vi "excel delete worksheet.vi"(8 "error in (no error)":errorcluster, 9 "Name of Worksheet to Delete":string="Sheet1", 10 "New worksheet":string="Intro", 11 "reference":T1) -> (0 "error out":errorcluster, 3 "reference out":T1)   [LabVIEW 2013]
doc: "Make a copy of active sheet. you can specify if the original is the active sheet \nafter the copy or the destination (copied sheet) should be active... \n\nYou need to supply a valid worksheet name (=destination), it should be unique \nwithin the workbook. to get a list of open sheets, use excel info.vi \n \nPhilips Research, COS/TMA"
uses:
  excel.llb/excel Object Reference.ctl
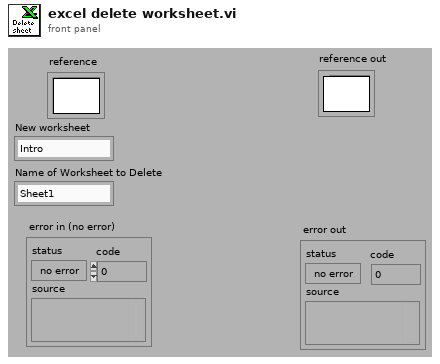
[diagram p1: front panel]
types:
  T1 = typedef "excel Object Reference.ctl" = refnum<k1>
  T2 = typedef "excel Data Members.ctl" = cluster{"Excel._Application":refnum<k7>, "Excel._Workbook":refnum<k7>, "Excel._Worksheet":refnum<k7>, "template?":bool, "location":cluster{"TopLeft":string, "RightBottom":string}, "positioning info":cluster{"direction":enum16{"right", "down"}, "gap":i32}}
  T3 = cluster{"direction":enum16{"right", "down"}, "gap":i32}
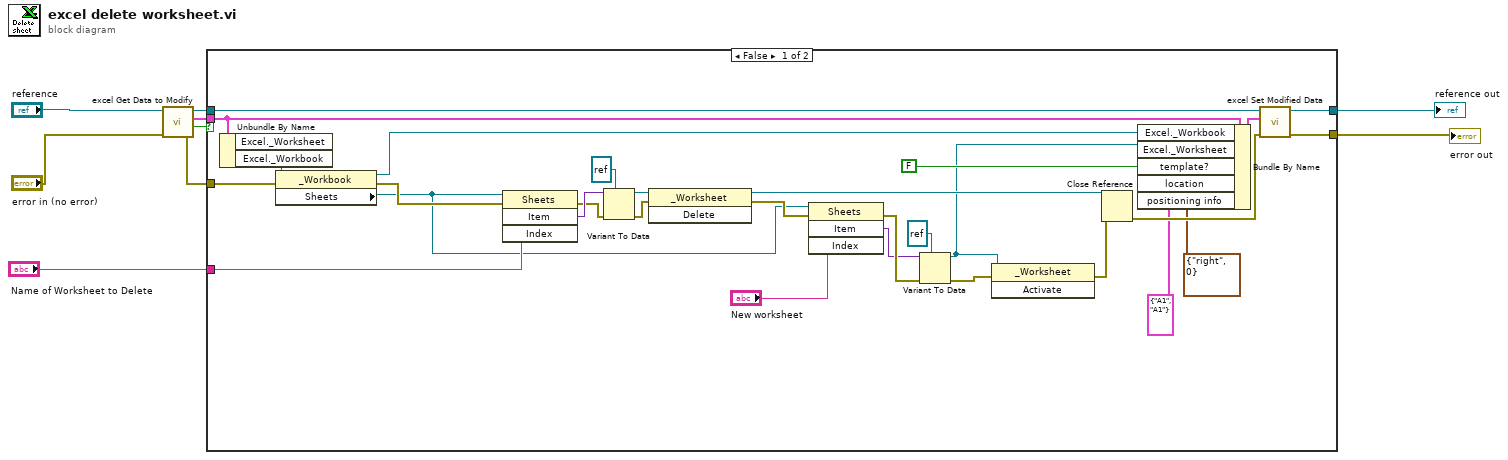
[diagram p0: block diagram]
diagram:
  n1 = call "excel Get Data to Modify.vi"("error in (no error)"="error in (no error)", "reference"="reference") -> ("error out"=w7:errorcluster, "timed out"=w8:bool, "data"=w9:T2, "duplicate reference"=w6:T1)  [unwired: 2 in]
  n2 = case shown="False" w8 {
    tunnel: w6 -> [w38 w39]
    tunnel: w9 -> [w20 _]
    tunnel: w7 -> [w37 w40]
    tunnel: [w36 w40] -> w3
    tunnel: [w35 w39] -> w4
    tunnel: "Name of Worksheet to Delete" -> [w26 _]
    frame False {
      n3 = Unbundle By Name(w20) -> ("Excel._Workbook"=w27:refnum<k7>)  [unwired: 1 out]
      n4 = property class="_Workbook"(reference=w27, error in=w37) -> (reference out=w17:refnum<k7>, error out=w30:errorcluster, "Sheets"=w24:refnum<k7>)
      n5 = invoke on="Invoke Node" class="Sheets" method="Item"(reference=w24, error in=w30, "Index"=w26) -> (error out=w32:errorcluster, "Item"=w34:variant)  [unwired: 1 in, 2 out]
      n6 = Variant To Data(error in=w32, type=refnum<k7> refnum ("Worksheets"), Variant=w34) -> (data=w33:refnum<k7>, error out=w31:errorcluster)
      n7 = invoke on="Invoke Node" class="_Worksheet" method="Delete"(reference=w33, error in=w31) -> (reference out=w28:refnum<k7>, error out=w25:errorcluster)  [unwired: 1 in, 1 out]
      n8 = invoke on="Invoke Node" class="Sheets" method="Item"(reference=w24, error in=w25, "Index"="New worksheet") -> (error out=w22:errorcluster, "Item"=w21:variant)  [unwired: 1 in, 2 out]
      n9 = Variant To Data(error in=w22, type=refnum<k7> refnum ("Worksheets"), Variant=w21) -> (data=w12:refnum<k7>, error out=w11:errorcluster)
      n10 = invoke class="_Worksheet" method="Activate"(reference=w12, error in=w11) -> (error out=w10:errorcluster)  [unwired: 1 in, 2 out]
      n11 = Close Reference(reference=w28, error in (no error)=w10) -> (error out=w18:errorcluster)
      n12 = Bundle By Name(cluster=w20, "Excel._Workbook"=w17, "Excel._Worksheet"=w12, "template?"=FALSE, "location"=cluster{"TopLeft":string, "RightBottom":string} {"TopLeft"="A1", "RightBottom"="A1"} ("Bundle Element"), "positioning info"=T3 {"direction"=enum."right", "gap"=0}) -> (w19:T2)
      n13 = call "excel Set Modified Data.vi"("error in (no error)"=w18, "data"=w19, "reference"=w38) -> ("error out"=w36:errorcluster, "duplicate reference"=w35:T1)  [unwired: 3 in]
    }
    frame True {
    }
  }
  "error out" <- w3
  "reference out" <- w4
